vi "write_with_ss.vi"(8 "Error in":errorcluster, 10 "power":dbl[](array[numeric]), 11 "temp":dbl[](array[numeric])) -> ()   [LabVIEW 2016]
uses:
  <vilib>/Utility/file.llb/Write Delimited Spreadsheet (DBL).vi
panel:
  in  "Header String":string
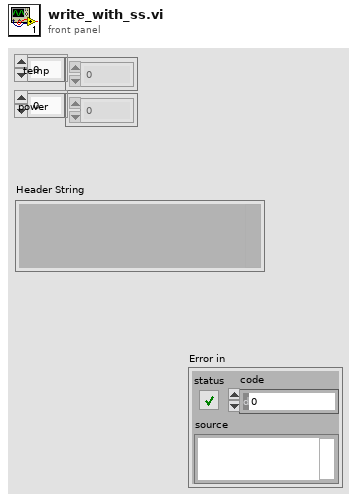
[diagram p1: front panel]
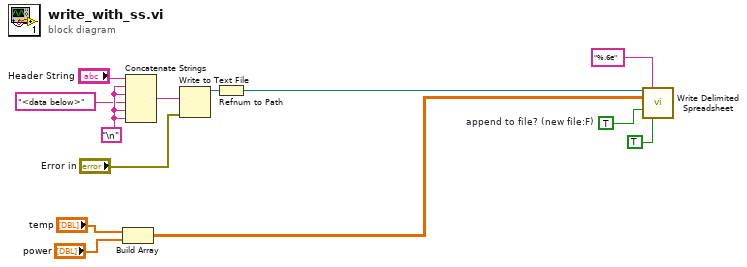
[diagram p0: block diagram]
diagram:
  w8 = TRUE  # append to file? (new file:F)
  w10 = "\n"
  n1 = Build Array("temp", "power") -> (w1:dbl[][])
  n2 = Concatenate Strings("Header String", w10, w10, "<data below>", w10, w10) -> (w7:string)
  n3 = Write to Text File(text=w7, error in="Error in") -> (refnum out=w6:refnum<file>)  [unwired: 2 in, 2 out]
  n4 = Refnum to Path(1:w6) -> (0:w5:path)
  n5 = call-poly <vilib>:"Write Delimited Spreadsheet.vi"("file path (dialog if empty)"=w5, "format (%.3f)"="%.6e", "2D data"=w1, "append to file? (new file:F)"=w8, "transpose? (no:F)"=TRUE ("Transpose Data?")) -> ()  [unwired: 9 in, 2 out]
